vi "Rocket Drive Immediate.vi"(4 "Right Joystick Y-Axis":dbl, 6 "Right Joystick X-Axis":dbl, 7 "Description":string, 8 "Command Info In":T1, 9 "Deadband Value":dbl=0.01, 10 "Left Joystick Y-Axis":dbl, 11 "Left Joystick X-Axis":dbl) -> (0 "Command Info Out":T1)   [LabVIEW 2020]
doc: "Often used for joystick control, this VI checks to see that the joystick axes are outside the deadband and updates the motors appropriately."
uses:
  <vilib>/Rock Robotics/WPI/Framework/Command Status Info.ctl
  <vilib>/Rock Robotics/WPI/Framework/Completion Status.ctl
  <vilib>/Rock Robotics/WPI/Framework/Completion Notifier.ctl
  Implementation/Drive Setpoints.ctl
  Implementation/Drive Operations.ctl
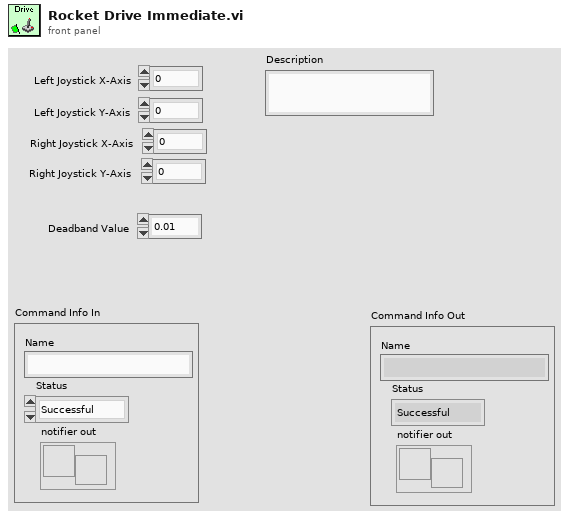
[diagram p1: front panel]
types:
  T1 = typedef "Command Status Info.ctl" = cluster{"Name":string, "Status":T2, "notifier out":T3}
  T2 = typedef "Completion Status.ctl" = enum16{"Successful", "Aborted", "Incomplete"}
  T3 = typedef "Completion Notifier.ctl" = refnum<notifier>
  T4 = typedef "Drive Setpoints.ctl" = cluster{"Operation":T5, "Left Joystick X-Axis":dbl, "Left Joystick Y-Axis":dbl, "Duration":dbl, "Right Joystick Y-Axis":dbl, "Right Joystick X-Axis":dbl}
  T5 = typedef "Drive Operations.ctl" = enum16{"Reserve", "Read Current", "Rocket Drive Immediate", "Tank Drive Immediate", "Drive for Time", "Drive for Distance"}
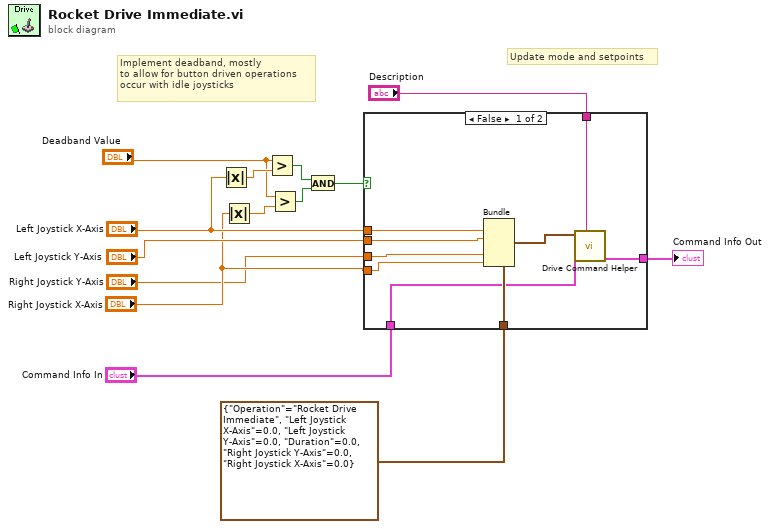
[diagram p0: block diagram]
diagram:
  # "Implement deadband, mostly\nto allow for button driven operations\noccur with idle joysticks"
  # "Update mode and setpoints"
  n1 = Absolute Value(x="Left Joystick X-Axis") -> (abs(x)=w14:dbl)
  n2 = Absolute Value(x="Right Joystick X-Axis") -> (abs(x)=w6:dbl)
  n3 = Greater?(x="Deadband Value", y=w14) -> (0:w8:bool)
  n4 = Greater?(x="Deadband Value", y=w6) -> (0:w5:bool)
  n5 = And(x=w8, y=w5) -> (x .and. y?=w7:bool)
  n6 = case shown="False" w7 {
    tunnel: "Left Joystick X-Axis" -> [w23 _]
    tunnel: T4 {"Operation"=enum."Rocket Drive Immediate", "Left Joystick X-Axis"=0.0, "Left Joystick Y-Axis"=0.0, "Duration"=0.0, "Right Joystick Y-Axis"=0.0, "Right Joystick X-Axis"=0.0} ("SubSystem Data") -> [w22 _]
    tunnel: [w21 w24] -> w13
    tunnel: "Command Info In" -> [w20 w24]
    tunnel: "Description" -> [w18 _]
    tunnel: "Right Joystick X-Axis" -> [w15 _]
    tunnel: "Left Joystick Y-Axis" -> [w17 _]
    tunnel: "Right Joystick Y-Axis" -> [w16 _]
    frame False {
      n7 = Bundle(cluster=w22, "Left Joystick X-Axis"=w23, "Left Joystick Y-Axis"=w17, "Right Joystick Y-Axis"=w16, "Right Joystick X-Axis"=w15) -> (w19:T4)  [unwired: 2 in]
      n8 = call "Drive Command Helper.vi"("Description"=w18, "Command Info In"=w20, "SubSystem Data"=w19) -> ("Command Info Out"=w21:T1)  [unwired: 6 in, 2 out]
    }
    frame True {
    }
  }
  "Command Info Out" <- w13
